vi "Read time end.vi"(8 "error in (no error)":errorcluster, 11 "Heater in":refnum<class "Heater_v2.lvclass">) -> (0 "error out":errorcluster, 2 "End":bool, 3 "Heater out":refnum<class "Heater_v2.lvclass">)   [LabVIEW 2019, in "Heater_v2.lvclass"]
uses:
  Heater_v2.lvclass
  Heater_v2.lvclass/Heater_v2.ctl
  REG/HE_reg.lvclass/HE_reg.ctl
  Reg/PID/PID SP Limiter/PID SP Limiter.lvclass/PID SP Limiter.ctl
  Reg/PID/PID SP Limiter/PID SP Limiter.lvclass
  REG/HE_reg.lvclass
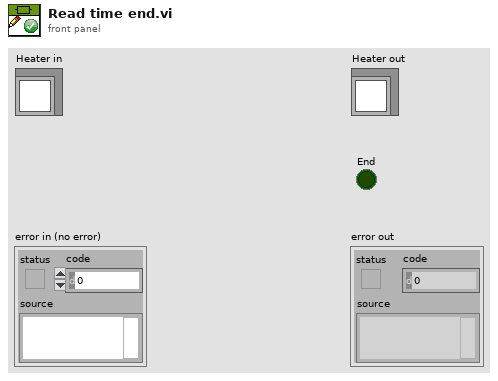
[diagram p1: front panel]
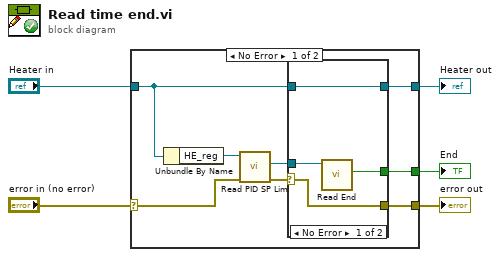
[diagram p0: block diagram]
diagram:
  n1 = case shown="No Error" "error in (no error)" {
    selector: "error in (no error)" -> [w7 w21]
    tunnel: [w11 w21] -> w4
    tunnel: [w12 w20] -> w2
    tunnel: "Heater in" -> [w13 w20]
    tunnel: [w10 _] -> w1
    frame No Error {
      n2 = Unbundle By Name(w13) -> ("HE_reg"=w6:refnum<class "HE_reg.lvclass">)
      n3 = call "Read PID SP Lim.vi"("error in (no error)"=w7, "HE_reg in"=w6) -> ("error out"=w8:errorcluster, "PID SP Limiter"=w9:refnum<class "PID SP Limiter.lvclass">)  [unwired: 7 in, 1 out]
      n4 = case shown="No Error" w8 {
        selector: w8 -> [w15 w18]
        tunnel: w13 -> [w16 w19]
        tunnel: [w16 w19] -> w12
        tunnel: [w15 w18] -> w11
        tunnel: w9 -> [w17 _]
        tunnel: [w14 _] -> w10
        frame No Error {
          n5 = call "Read End.vi"("PID SP Limiter in"=w17) -> ("End"=w14:bool)  [unwired: 9 in, 1 out]
        }
        frame Error {
        }
      }
    }
    frame Error {
    }
  }
  "error out" <- w4
  "Heater out" <- w2
  "End" <- w1
